vi "Set Wideband AC Voltage.vi"(8 "error in (no error)":errorcluster, 10 "Wideband Mode (F: Off)":bool, 11 "VISA resource name":refnum<visa-resource-name>) -> (0 "error out":errorcluster {"code" format="%.0x"}, 3 "VISA resource name out":refnum<visa-resource-name>)   [LabVIEW 2014, in "Fluke 5XXX Series Multicalibrators.lvlib"]
doc: "This VI activates or deactivates output from the Wideband AC Module (Option 5700A-03).\n\nNote:\n\nThis VI is available only for instrument models 5700A and 5720A with option 5700A-03."
uses:
  Fluke 5XXX Series Multicalibrators.lvlib
panel:
  # "On"
  # "Off"
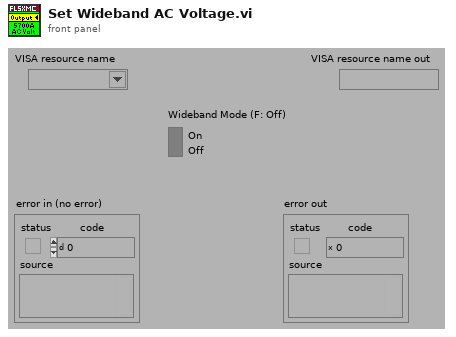
[diagram p1: front panel]
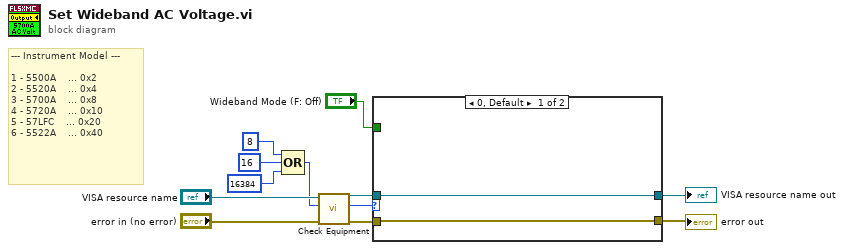
[diagram p0: block diagram]
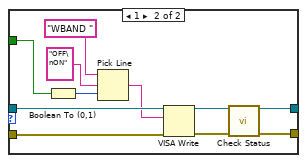
[diagram p2: hidden frame]
diagram:
  # "--- Instrument Model ---\n\n1 - 5500A    ... 0x2\n2 - 5520A    ... 0x4\n3 - 5700A    ... 0x8\n4 - 5720A    ... 0x10\n5 - 57LFC    ... 0x20\n6 - 5522A    ... 0x40"
  n1 = Compound Arithmetic op=OR(8 ("Numeric"), 16 ("Numeric"), 16384 ("Numeric")) -> (w5:i32)
  n2 = call "Check Equipment.vi"("error in (no error)"="error in (no error)", "Bit Mask"=w5, "VISA resource name"="VISA resource name") -> ("error out"=w12:errorcluster, "Present?"=w11:u32, "VISA resource name out"=w10:refnum<visa-resource-name>)  [unwired: 6 in]
  n3 = case shown="0, Default" w11 {
    tunnel: "Wideband Mode (F: Off)" -> [_ w22]
    tunnel: [w13 w16] -> w1
    tunnel: w12 -> [w14 w21]
    tunnel: w10 -> [w13 w20]
    tunnel: [w14 w17] -> w2
    frame 0, Default {
    }
    frame 1 {
      n4 = Boolean To (0,1)(Boolean=w22) -> (0, 1=w23:i16)
      n5 = Pick Line(string ("")="WBAND " ("Reset Command"), multi-line string="OFF\nON", line index=w23) -> (output string=w19:string)
      n6 = VISA Write(VISA resource name=w20, write buffer=w19, error in (no error)=w21) -> (VISA resource name out=w15:refnum<visa-resource-name>, error out=w18:errorcluster)  [unwired: 1 out]
      n7 = call "Check Status.vi"("VISA resource name"=w15, "error in (no error)"=w18) -> ("VISA resource name out"=w16:refnum<visa-resource-name>, "error out"=w17:errorcluster)  [unwired: 12 in]
    }
  }
  "VISA resource name out" <- w1
  "error out" <- w2
